vi "Stand alove FP.vi"() -> ()   [LabVIEW 2015]
panel:
  out "Thermometer":dbl(slide) scale=0.0..100.0
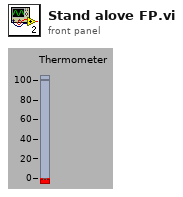
[diagram p1: front panel]
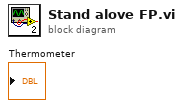
[diagram p0: block diagram]
diagram:
